vi "CS-4 Get Sweep Mode.vi"(4 "error in (no error)":errorcluster, 7 "VISA session":refnum<visa-resource-name>) -> (0 "error out":errorcluster, 1 "sweep mode":T1, 2 "response out":string, 3 "dup VISA session":refnum<visa-resource-name>)   [LabVIEW 2020]
doc: "CS-4 Get Sweep Mode.vi will return the present power supply sweep mode (sweep up, zero,sweep down, fast) as a boolean indicator cluster. The text string from the instrument will also be returned unmodified."
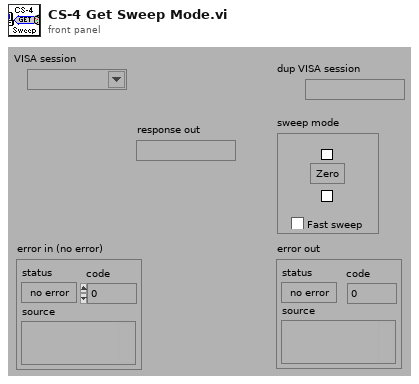
[diagram p1: front panel]
types:
  T1 = cluster{"zero":bool, "sweep up":bool, "sweep down":bool, "fast sweep":bool}
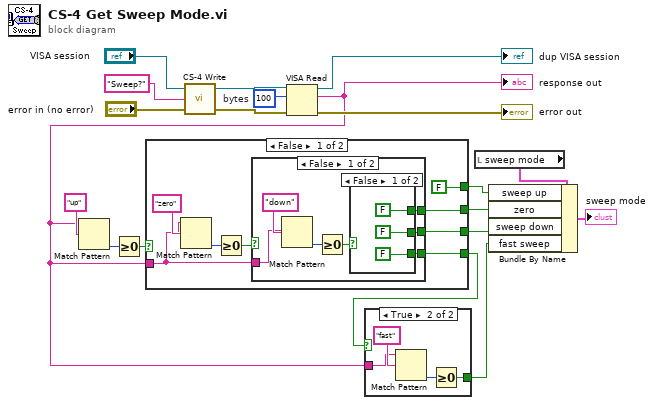
[diagram p0: block diagram]
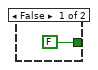
[diagram p2: hidden frame]
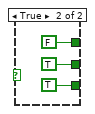
[diagram p3: hidden frame]
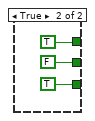
[diagram p4: hidden frame]
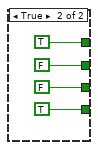
[diagram p5: hidden frame]
diagram:
  w14 = u32 100  # bytes
  n1 = call "CS-4 Write.vi"("error in (no error)"="error in (no error)", "write buffer (\"\")"="Sweep?", "VISA session"="VISA session") -> ("error out"=w16:errorcluster, "dup VISA session"=w17:refnum<visa-resource-name>)  [unwired: 1 out]
  n2 = VISA Read(VISA resource name=w17, byte count=w14, error in (no error)=w16) -> (VISA resource name out=→"dup VISA session":refnum<visa-resource-name>, read buffer=w8:string, error out=→"error out":errorcluster)  [unwired: 1 out]
  "response out" <- w8
  n3 = Match Pattern(string=w8, regular expression="up") -> (offset past match=w11:i32)  [unwired: 1 in, 3 out]
  n4 = Greater Or Equal To 0?(x=w11) -> (x >= 0?=w10:bool)
  n5 = case shown="False" w10 {
    tunnel: w8 -> [w24 _]
    tunnel: [w23 FALSE] -> w6
    tunnel: [w22 TRUE] -> w7
    tunnel: [w21 FALSE] -> w5
    tunnel: [FALSE TRUE] -> w4
    frame False {
      n6 = Match Pattern(string=w24, regular expression="zero") -> (offset past match=w27:i32)  [unwired: 1 in, 3 out]
      n7 = Greater Or Equal To 0?(x=w27) -> (x >= 0?=w25:bool)
      n8 = case shown="False" w25 {
        tunnel: w24 -> [w32 _]
        tunnel: [w29 FALSE] -> w23
        tunnel: [w28 TRUE] -> w22
        tunnel: [w30 TRUE] -> w21
        frame False {
          n9 = Match Pattern(string=w32, regular expression="down") -> (offset past match=w33:i32)  [unwired: 1 in, 3 out]
          n10 = Greater Or Equal To 0?(x=w33) -> (x >= 0?=w31:bool)
          n11 = case shown="False" w31 {
            tunnel: [FALSE FALSE] -> w30
            tunnel: [FALSE TRUE] -> w29
            tunnel: [FALSE TRUE] -> w28
            frame False {
            }
            frame True {
            }
          }
        }
        frame True {
        }
      }
    }
    frame True {
    }
  }
  n12 = case shown="True" w7 {
    tunnel: w8 -> [_ w50]
    tunnel: [FALSE w49] -> w3
    frame False {
    }
    frame True {
      n13 = Match Pattern(string=w50, regular expression="fast") -> (offset past match=w51:i32)  [unwired: 1 in, 3 out]
      n14 = Greater Or Equal To 0?(x=w51) -> (x >= 0?=w49:bool)
    }
  }
  n15 = local read "sweep mode"() -> (w1:T1)
  n16 = Bundle By Name(cluster=w1, "sweep up"=w4, "zero"=w5, "sweep down"=w6, "fast sweep"=w3) -> (→"sweep mode":T1)
